vi "Restart Relay Blue TSFTS2.vi"(8 "error in (no error)":errorcluster) -> (0 "error out":errorcluster, 1 "Result (bool)":bool, 3 "VISA resource OUT":refnum<visa-resource-name>)   [LabVIEW 2022 SP3]
uses:
  <vilib>/DAQmx/write.llb/DAQmx Write (Digital Bool 1Line 1Point).vi
  <vilib>/DAQmx/miscellaneous.llb/DAQmx Fill In Error Info.vi
panel:
  out "Instructional Message":string="Did the control power turn off?"
  in  "No":bool
  in  "Yes":bool
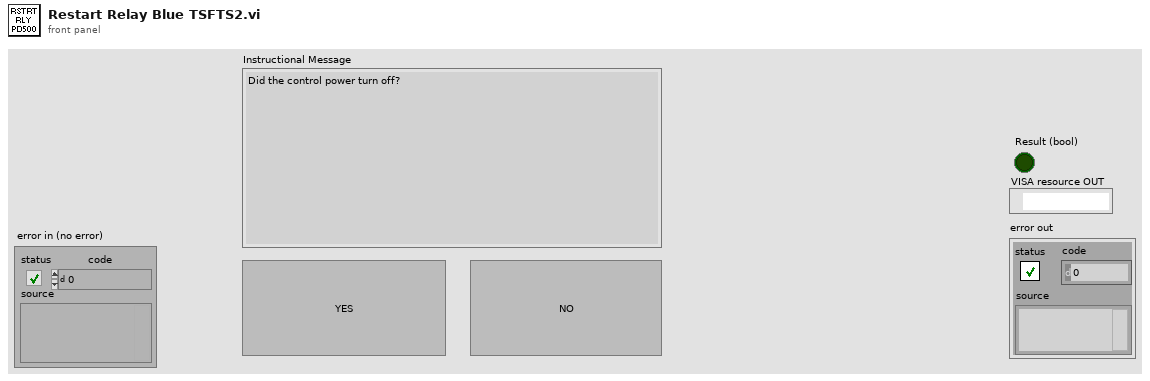
[diagram p1: front panel]
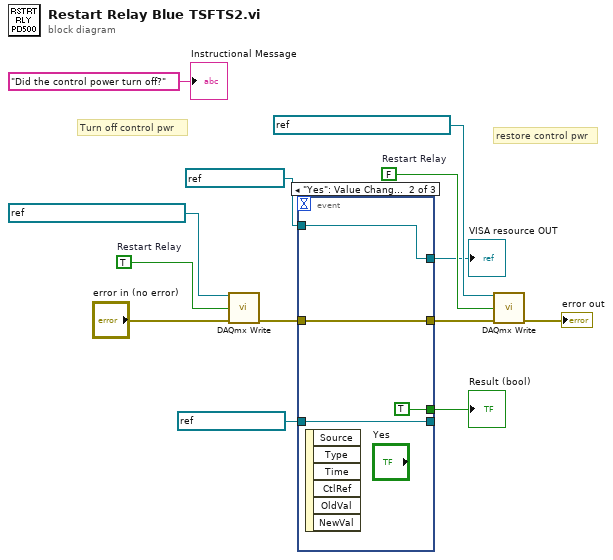
[diagram p0: block diagram]
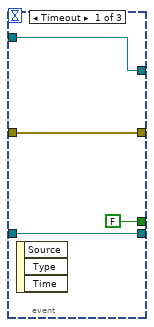
[diagram p2: hidden frame]
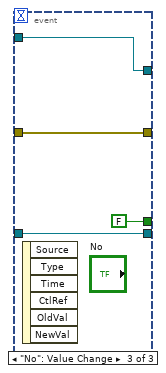
[diagram p3: hidden frame]
diagram:
  w9 = TRUE  # Restart Relay
  w11 = FALSE  # Restart Relay
  # "restore control pwr"
  # "Turn off control pwr"
  n1 = call-poly <vilib>:"DAQmx Write.vi"("task/channels in"=refnum<k21> "FTS2_PD500_ProgramRestart", "data"=w9, "error in"="error in (no error)") -> ("error out"=w7:errorcluster)  [unwired: 10 in, 2 out]
  n2 = event shown="[1] \"Yes\": Value Change" {
    selector: _ -> [_ _ _]
    dyn-events: _ -> [_ _ _]
    timeout: _ -> [_ _ _]
    tunnel: [FALSE TRUE FALSE] -> w5
    tunnel: w7 -> [w17 w20 w24]
    tunnel: [w17 w20 w24] -> w6
    tunnel: refnum<visa-resource-name> "ControlBoard" ("VISA resource name") -> [w16 w19 w23]
    tunnel: [w16 w19 w23] -> w4
    tunnel: [w14 w18 w22] -> _
    tunnel: refnum<visa-resource-name> "HMP4040_FTS2" ("HMP4040 IN") -> [w14 w18 w22]
    event Timeout {
      n3 = event-data() -> ()  [unwired: 1 in, 3 out]
    }
    event "Yes": Value Change {
      n4 = event-data() -> ()  [unwired: 1 in, 6 out]
    }
    event "No": Value Change {
      n5 = event-data() -> ()  [unwired: 1 in, 6 out]
    }
  }
  "VISA resource OUT" <- w4
  "Result (bool)" <- w5
  n6 = call-poly <vilib>:"DAQmx Write.vi"("task/channels in"=refnum<k21> "FTS2_PD500_ProgramRestart", "data"=w11, "error in"=w6) -> ("error out"=→"error out":errorcluster)  [unwired: 10 in, 2 out]
  "Instructional Message" <- "Did the control power turn off?" ("Instructional Message")
